vi "SwitchMechanicalActions.vi"() -> ()   [LabVIEW 2020]
panel:
  in  "Reset":bool
  out "Time (sec) 6":dbl
  out "Time (sec) 4":dbl
  out "Time (sec) 5":dbl
  out "Time (sec) 3":dbl
  out "Time (sec) 2":dbl
  out "Time (sec) 1":dbl
  in  "Stop":bool
  out "LED 6":bool
  out "LED 5":bool
  out "LED 4":bool
  out "LED 3":bool
  out "LED 2":bool
  out "LED 1":bool
  in  "Latch until released":bool
  in  "Latch when released":bool
  in  "Latch when pressed":bool
  in  "Switch until released":bool
  in  "Switch when released":bool
  in  "Switch when pressed":bool
  # "Shows how much time the button is in on state."
  # "Instructions:\n1. Press the reset button to make all the values to zero.\n2. Press the \"Stop\" button to stop the program."
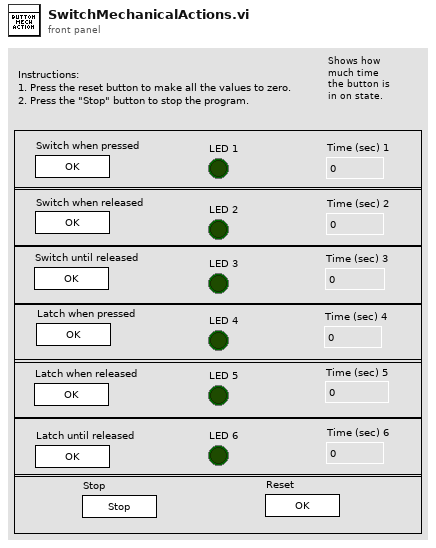
[diagram p1: front panel]
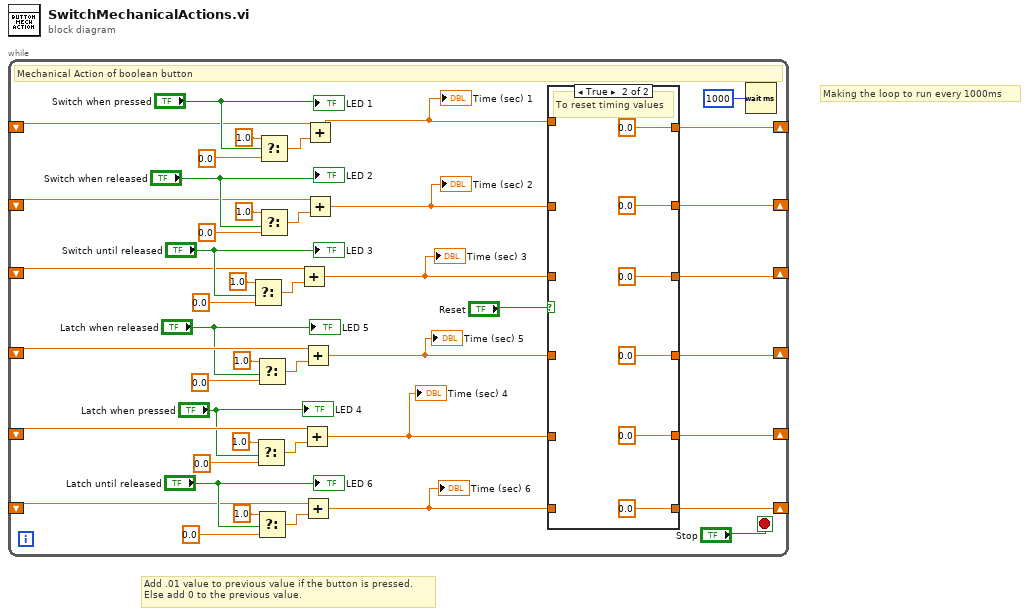
[diagram p0: block diagram]
diagram:
  # "Making the loop to run every 1000ms"
  # "Add .01 value to previous value if the button is pressed.\nElse add 0 to the previous value."
  n1 = while {
    shift-right: [w20] -> _
    shift-left: _ -> [w11]
    shift-right: [w18] -> _
    shift-left: _ -> [w10]
    shift-right: [w16] -> _
    shift-left: _ -> [w9]
    shift-right: [w15] -> _
    shift-left: _ -> [w8]
    shift-right: [w14] -> _
    shift-left: _ -> [w7]
    shift-right: [w12] -> _
    shift-left: _ -> [w6]
    stop <- "Stop" stop-if-true
    # "Mechanical Action of boolean button"
    n2 = Select(t=1.0, s="Switch until released", f=0.0) -> (s? t:f=w37:dbl)
    n3 = Select(t=1.0, s="Latch when pressed", f=0.0) -> (s? t:f=w30:dbl)
    n4 = Select(t=1.0, s="Latch when released", f=0.0) -> (s? t:f=w33:dbl)
    n5 = Select(t=1.0, s="Latch until released", f=0.0) -> (s? t:f=w27:dbl)
    n6 = Select(t=1.0, s="Switch when pressed", f=0.0) -> (s? t:f=w44:dbl)
    n7 = Select(t=1.0, s="Switch when released", f=0.0) -> (s? t:f=w40:dbl)
    n8 = Add(x=w9, y=w37) -> (x+y=w17:dbl)
    "Time (sec) 3" <- w17
    n9 = Add(x=w7, y=w30) -> (x+y=w1:dbl)
    "Time (sec) 4" <- w1
    n10 = Add(x=w8, y=w33) -> (x+y=w2:dbl)
    "Time (sec) 5" <- w2
    n11 = Add(x=w6, y=w27) -> (x+y=w13:dbl)
    "Time (sec) 6" <- w13
    n12 = Add(x=w11, y=w44) -> (x+y=w21:dbl)
    "Time (sec) 1" <- w21
    n13 = Add(x=w10, y=w40) -> (x+y=w19:dbl)
    "Time (sec) 2" <- w19
    n14 = case shown="True" "Reset" {
      tunnel: w21 -> [w51 _]
      tunnel: [w51 0.0] -> w20
      tunnel: w19 -> [w50 _]
      tunnel: [w50 0.0] -> w18
      tunnel: [w49 0.0] -> w16
      tunnel: w17 -> [w49 _]
      tunnel: [w48 0.0] -> w15
      tunnel: w2 -> [w48 _]
      tunnel: [w47 0.0] -> w14
      tunnel: w1 -> [w47 _]
      tunnel: [w46 0.0] -> w12
      tunnel: w13 -> [w46 _]
      frame False {
      }
      frame True {
        # "To reset timing values"
      }
    }
    n15 = Wait (ms)(milliseconds to wait=u32 1000) -> ()  [unwired: 1 out]
    "LED 1" <- "Switch when pressed"
    "LED 2" <- "Switch when released"
    "LED 3" <- "Switch until released"
    "LED 4" <- "Latch when pressed"
    "LED 5" <- "Latch when released"
    "LED 6" <- "Latch until released"
  }
